vi "PC_decimate_waveform.vi"(8 "error in (no error)":errorcluster, 10 "decimating factor":i32, 11 "Waveform in":waveform(dbl)) -> (0 "error out":errorcluster, 3 "Waveform out":waveform(dbl))   [LabVIEW 2020]
uses:
  <vilib>/Analysis/2dsp.llb/Decimate (continuous, DBL).vi
  <vilib>/Analysis/NI_AALPro.lvlib
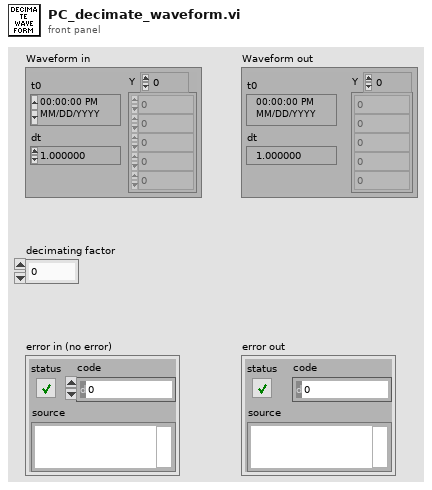
[diagram p1: front panel]
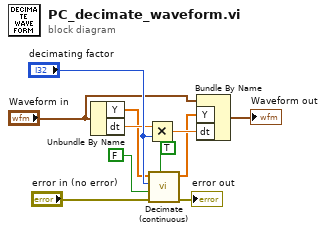
[diagram p0: block diagram]
diagram:
  n1 = Unbundle By Name("Waveform in") -> ("Y"=w2:dbl[], "dt"=w6:dbl)
  n2 = Multiply(x=w6, y="decimating factor") -> (x*y=w8:dbl)
  n3 = call-poly <vilib>:"Decimate (continuous).vi"("reset"=TRUE, "error in (no error)"="error in (no error)", "averaging"=FALSE, "decimating factor"="decimating factor", "X"=w2) -> ("error out"=→"error out":errorcluster, "Decimated Array"=w4:dbl[])  [unwired: 5 in]
  n4 = Bundle By Name(cluster="Waveform in", "Y"=w4, "dt"=w8) -> (→"Waveform out":waveform(dbl))
